vi "test1.vi"() -> ()   [LabVIEW 2013]
uses:
  <vilib>/Platform/TimedLoop/XDataNode/timing_clust.ctl
  <vilib>/Platform/TimedLoop/XDataNode/nitl_modes.ctl
  <vilib>/Platform/TimedLoop/XDataNode/wakeup.ctl
  <vilib>/platform/TimedLoop/XDataNode/XDataNode.xnode
  <vilib>/Platform/TimedLoop/XDataNode/XDNodeRunTimeDep.lvlib
panel:
  out "String":string
  out "Boolean":bool
  in  "OK Button":bool
  in  "stop":bool
  out "Numeric":dbl
  out "error out":errorcluster
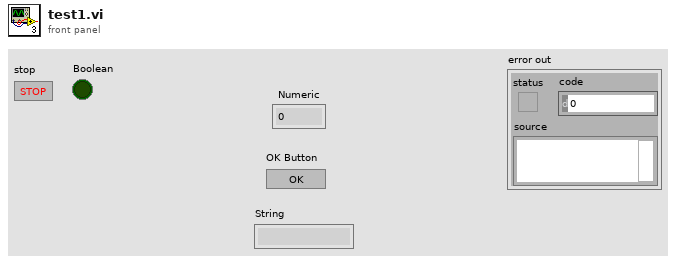
[diagram p1: front panel]
types:
  T1 = typedef "XDNodeRunTimeDep.lvlib/timing_clust.ctl" = cluster{"Expected End [f-1]":u64, "Actual End [f-1]":u64, "Finished Late? [f-1]":bool, "Expected End [i-1]":u64, "Actual End [i-1]":u64, "Finished Late? [i-1]":bool, "Expected Start [i]":u64, "Actual Start [i]":u64, "Expected Start [f]":u64, "Actual Start [f]":u64, "Source Name":string, "Structure Name":string, "Period":i64, "Deadline":i64, "Offset":i64, "Start":i64, "Priority":i32, "Timeout":i32, "Mode":T2, "Wakeup Reason":T3, "Error":errorcluster, "Source Type":string, "Secondary Source Type":string, "Global End Time":u64, "Global Start Time":u64, "Frame Duration":u64, "Iteration Duration":u64, "Assigned CPU":i32, "I/O Scan Engine Mode":u32}
  T2 = typedef "XDNodeRunTimeDep.lvlib/nitl_modes.ctl" = enum32{"No Change", "Process missed periods, maintain original phase", "Discard missed periods, maintain original phase", "Process missed periods, ignore original phase", "Discard missed periods, ignore original phase"}
  T3 = typedef "XDNodeRunTimeDep.lvlib/wakeup.ctl" = enum32{"Normal", "Aborted", "Asynchronous wakeup", "Timing source error", "Timed loop error", "Timeout"}
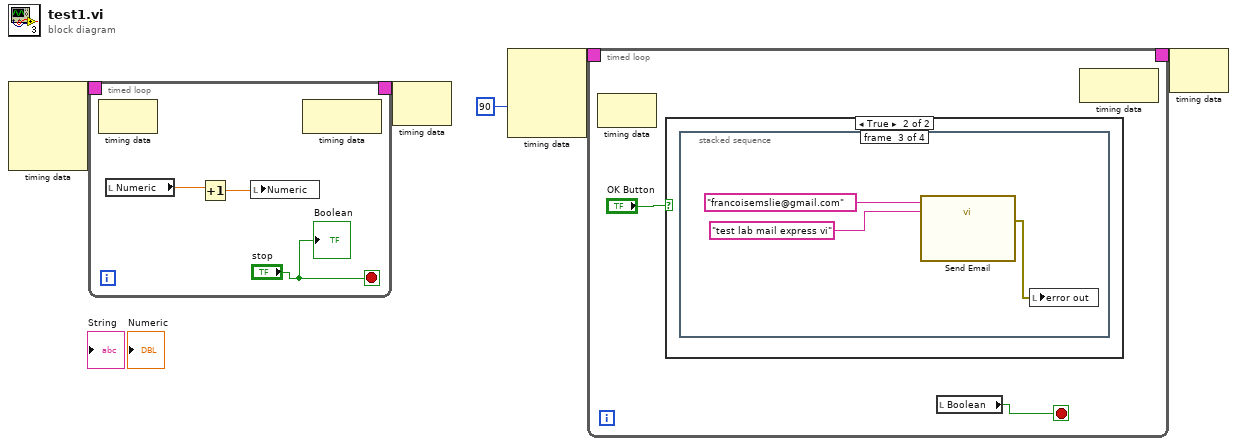
[diagram p0: block diagram]
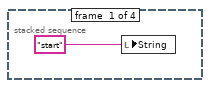
[diagram p3: hidden frame]
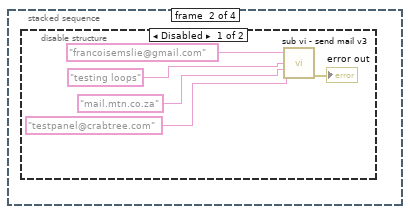
[diagram p4: hidden frame]
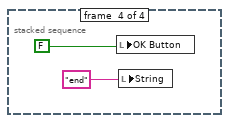
[diagram p6: hidden frame]
diagram:
  n1 = node-c288() -> (w5:T1)  [unwired: 4 in]
  n2 = timed-loop {
    timing: w5 -> [_]
    timing-out: [_] -> w4
    stop <- "stop" stop-if-true
    n3 = node-c288() -> ()  [unwired: 1 in, 1 out]
    n4 = local read "Numeric"() -> (w8:dbl)
    n5 = Increment(x=w8) -> (x+1=w7:dbl)
    n6 = local write "Numeric"(w7) -> ()
    n7 = node-c288() -> ()  [unwired: 1 in, 1 out]
    "Boolean" <- "stop"
  }
  n8 = node-c288(w4) -> ()  [unwired: 1 out]
  n9 = node-c288(90) -> (w3:T1)  [unwired: 3 in]
  n10 = timed-loop {
    timing: w3 -> [_]
    timing-out: [_] -> w2
    stop <- w11 stop-if-true
    n11 = node-c288() -> ()  [unwired: 1 in, 1 out]
    n12 = case shown="True" "OK Button" {
      frame False {
      }
      frame True {
        n13 = stacked-sequence {
          frame #0 {
            n14 = local write "String"("start") -> ()
          }
          frame #1 {
            n15 = disable-structure shown="Disabled" {
              frame Disabled {
                n16 = call "sub vi - send mail v3.vi"("TO:"="francoisemslie@gmail.com", "subject"="testing loops", "out going server"="mail.mtn.co.za", "from"="testpanel@crabtree.com") -> ("error out"=→"error out":errorcluster)  [unwired: 11 in]
              }
              frame Enabled {
              }
            }
          }
          frame #2 {
            n17 = call "Send Email"("Subject"="test lab mail express vi", "Recipients"="francoisemslie@gmail.com") -> ("error out"=w21:errorcluster)  [unwired: 9 in]
            n18 = local write "error out"(w21) -> ()
          }
          frame #3 {
            n19 = local write "OK Button"(FALSE) -> ()
            n20 = local write "String"("end") -> ()
          }
        }
      }
    }
    n21 = local read "Boolean"() -> (w11:bool)
    n22 = node-c288() -> ()  [unwired: 1 in, 1 out]
  }
  n23 = node-c288(w2) -> ()  [unwired: 1 out]
